vi "CANtest2.vi"() -> ()   [LabVIEW 2017]
uses:
  <vilib>/addons/Maxon Motor/EPOS2 CANopen/EPOS2 Support Files/Typedefs/EPOS2 Status Word PVM.ctl
  <vilib>/addons/Maxon Motor/EPOS2 CANopen/EPOS2 Support Files/Typedefs/EPOS2 Data Output Current.ctl
  <vilib>/addons/Maxon Motor/EPOS2 CANopen/CANopen/sbCANopenBaseClass.lvclass
  <vilib>/addons/Maxon Motor/EPOS2 CANopen/EPOS2 Support Files/Typedefs/EPOS2 Control Word PVM.ctl
  <vilib>/Platform/TimedLoop/XDataNode/timing_clust.ctl
  <vilib>/Platform/TimedLoop/XDataNode/nitl_modes.ctl
  <vilib>/Platform/TimedLoop/XDataNode/wakeup.ctl
  <vilib>/Platform/TimedLoop/XDataNode/XDataNode.xnode
  <vilib>/Platform/TimedLoop/XDataNode/XDNodeRunTimeDep.lvlib
  <vilib>/addons/Maxon Motor/EPOS2 CANopen/EPOS2 Library.lvlib
  <vilib>/addons/Maxon Motor/EPOS2 CANopen/EPOS2 Support Files/Polymorphic SubVIs/Read PDO/EPOS2 Current Mode Read.vi
  <vilib>/addons/Maxon Motor/EPOS2 CANopen/EPOS2 Support Files/Polymorphic SubVIs/Write PDO/EPOS2 Current Mode Write.vi
panel:
  out "nmotors":i32=4
  out "Velocity 2":i32[](array[numeric])
  out "Array":refnum<class "sbCANopenBaseClass.lvclass">[](array[class])
  in  "Current":i32=10
  out "Velocity":i32[](array[numeric])
  out "I32":i32
  out "Data Output 5":T1
  out "Data Output 4":T1
  out "Data Output 3":T1
  out "Data Output":T1
  out "Array 3":u8[](array[numeric])
  out "Iteration Duration 3":i64
  out "Read Late":bool
  in  "Array 2":dbl[](array[numeric])=[500.0, 600.0, 300.0, 0.0]
  out "Statusword":T2={"Ready to Switch On"=TRUE, "Switched On"=TRUE, "Operation Enable"=TRUE, "Fault"=FALSE, "Voltage Enabled"=TRUE, "Quick Stop"=TRUE, "Switch On Disable"=FALSE, "Warning"=FALSE, "Offset Current Measured"=TRUE, "Remote"=FALSE, "Target Reached"=FALSE, "Internal Limit Active"=FALSE, "Speed"=FALSE, "Reserved"=FALSE, "Refresh Cycle of Power Stage"=FALSE, "Position Reference to Home Position"=FALSE}
  out "Node":i32
  out "During Automatic":T2
  in  "STOP Final":bool
  out "Iteration Duration":i64
  in  "stop":bool
  in  "Current 2":i32(slide) scale=-1000.0..1000.0
  out "Node ID 3":u8
  in  "motor #":i32
  in  "Switch On":bool=TRUE
  in  "motor enable":i32
  in  "enable ready 2":bool
  out "Finished Late? [i-1] 3":bool
  out "Numeric 3":i32
  out "Iteration Duration 2":i64
  out "Write Late":bool
  out "Node ID\nin while loop 2":u8
  out "Node ID\nin while loop":u8
  out "for 1":i32
  # "reading purposes"
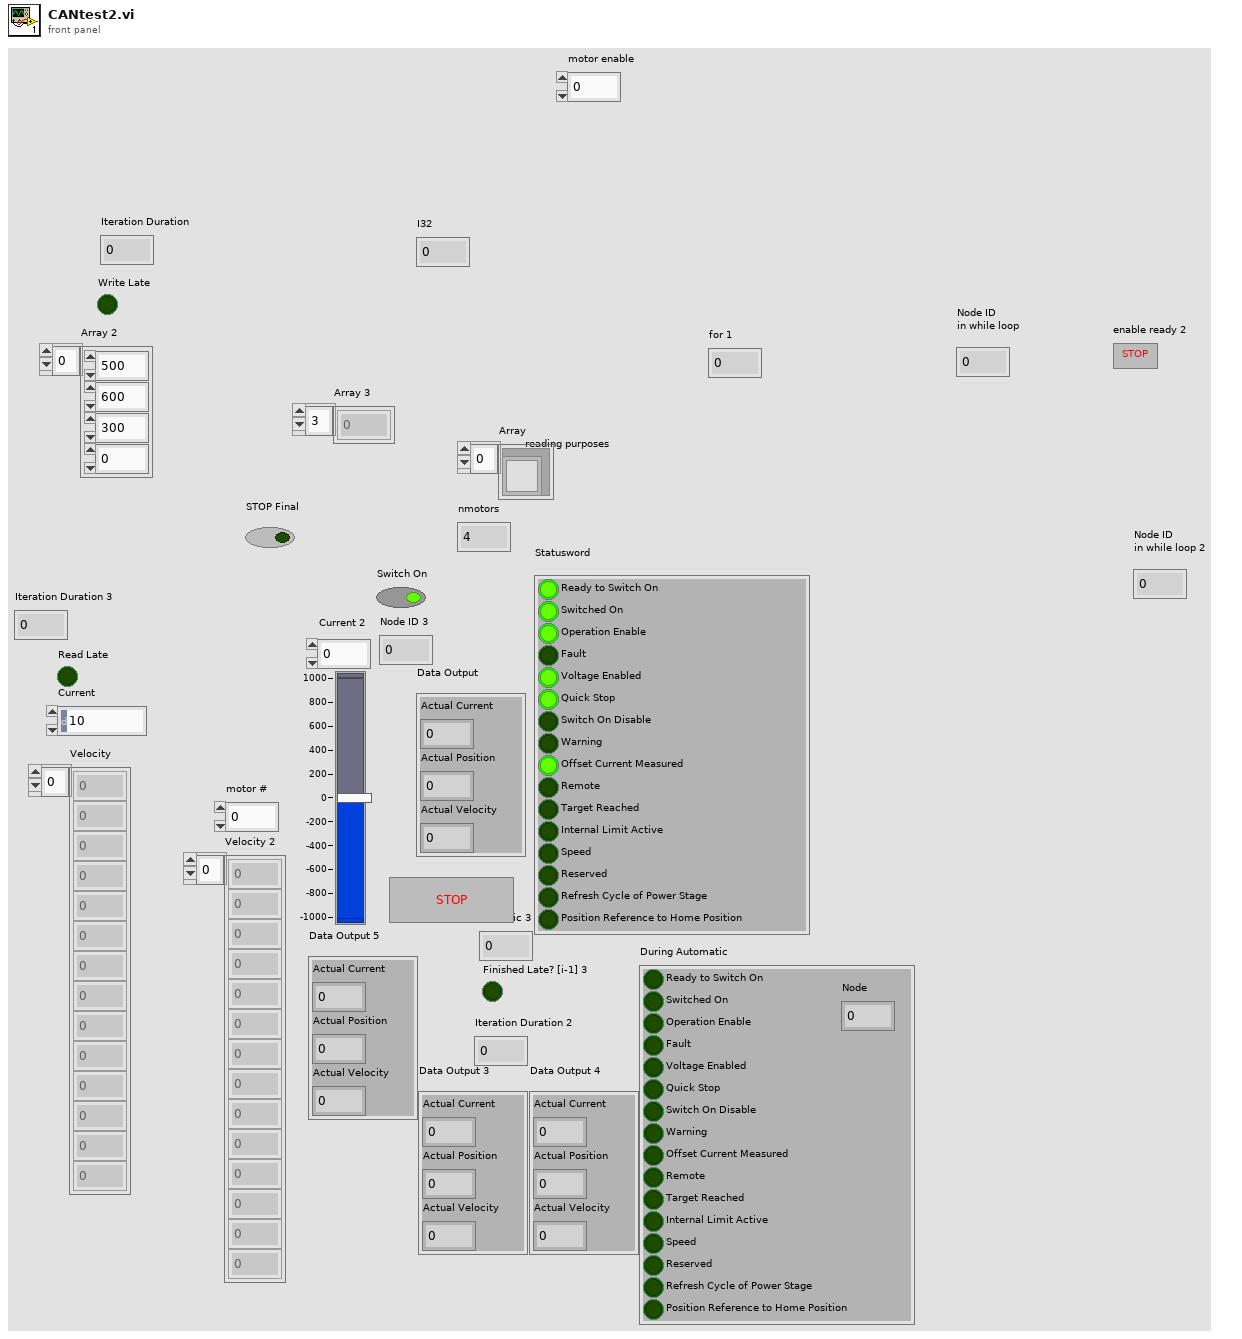
[diagram p1: front panel]
types:
  T1 = typedef "EPOS2 Library.lvlib/EPOS2 Data Output Current.ctl" = cluster{"Actual Current":i16, "Actual Position":i32, "Actual Velocity":i32}
  T2 = typedef "EPOS2 Library.lvlib/EPOS2 Status Word PVM.ctl" = cluster{"Ready to Switch On":bool, "Switched On":bool, "Operation Enable":bool, "Fault":bool, "Voltage Enabled":bool, "Quick Stop":bool, "Switch On Disable":bool, "Warning":bool, "Offset Current Measured":bool, "Remote":bool, "Target Reached":bool, "Internal Limit Active":bool, "Speed":bool, "Reserved":bool, "Refresh Cycle of Power Stage":bool, "Position Reference to Home Position":bool}
  T3 = typedef "XDNodeRunTimeDep.lvlib/timing_clust.ctl" = cluster{"Expected End [f-1]":u64, "Actual End [f-1]":u64, "Finished Late? [f-1]":bool, "Expected End [i-1]":u64, "Actual End [i-1]":u64, "Finished Late? [i-1]":bool, "Expected Start [i]":u64, "Actual Start [i]":u64, "Expected Start [f]":u64, "Actual Start [f]":u64, "Source Name":string, "Structure Name":string, "Period":i64, "Deadline":i64, "Offset":i64, "Start":i64, "Priority":i32, "Timeout":i32, "Mode":T4, "Wakeup Reason":T5, "Error":errorcluster, "Source Type":string, "Secondary Source Type":string, "Global End Time":u64, "Global Start Time":u64, "Frame Duration":u64, "Iteration Duration":u64, "Assigned CPU":i32, "I/O Scan Engine Mode":u32}
  T4 = typedef "XDNodeRunTimeDep.lvlib/nitl_modes.ctl" = enum32{"No Change", "Process missed periods, maintain original phase", "Discard missed periods, maintain original phase", "Process missed periods, ignore original phase", "Discard missed periods, ignore original phase"}
  T5 = typedef "XDNodeRunTimeDep.lvlib/wakeup.ctl" = enum32{"Normal", "Aborted", "Asynchronous wakeup", "Timing source error", "Timed loop error", "Timeout"}
  T6 = typedef "EPOS2 Library.lvlib/EPOS2 Control Word PVM.ctl" = cluster{"Switch On":bool, "Enable Voltage":bool, "Quick Stop":bool, "Enable Operation":bool, "Reserved 0":bool, "Reserved 1":bool, "Reserved 2":bool, "Fault Reset":bool, "Halt":bool}
  T7 = cluster{"[0]":bool, "[1]":bool, "[2]":bool, "[3]":bool, "[4]":bool, "[5]":bool, "[6]":bool, "[7]":bool, "[8]":bool, "[9]":bool, "[10]":bool, "[11]":bool, "[12]":bool, "[13]":bool, "[14]":bool, "[15]":bool}
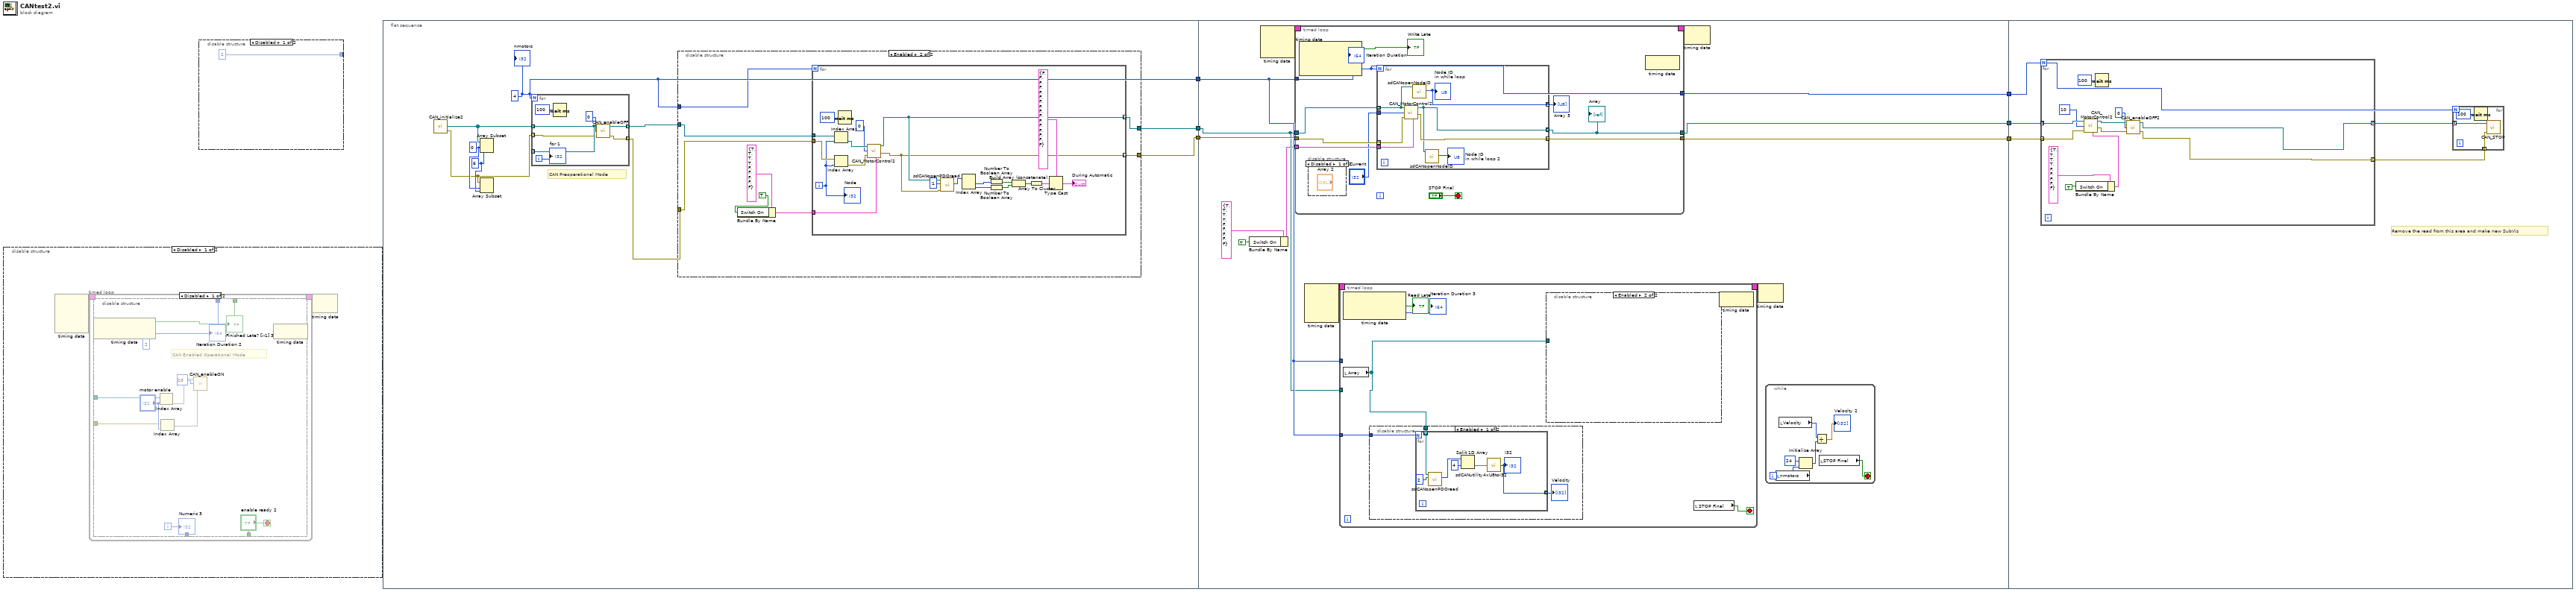
[diagram p0: block diagram]
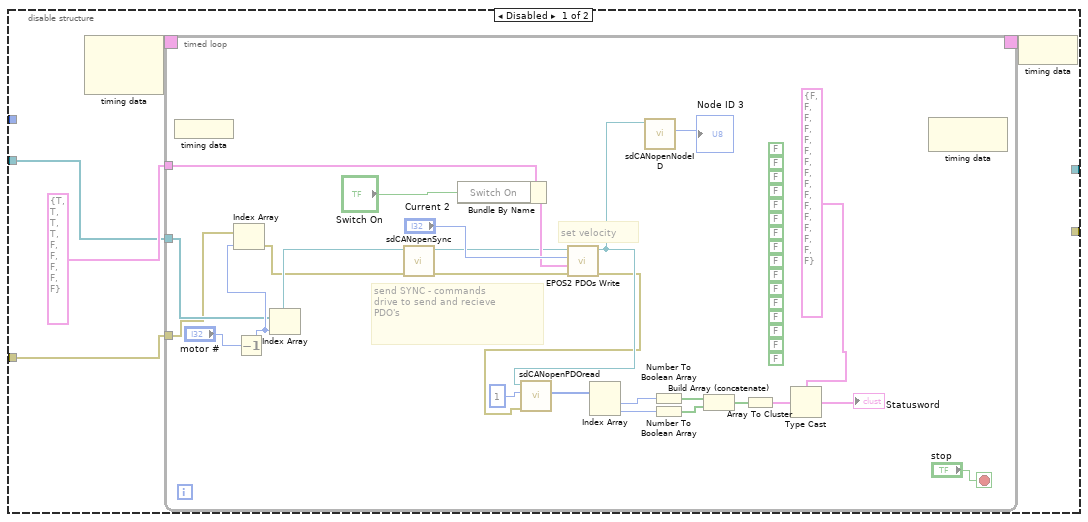
[diagram p5: hidden frame]
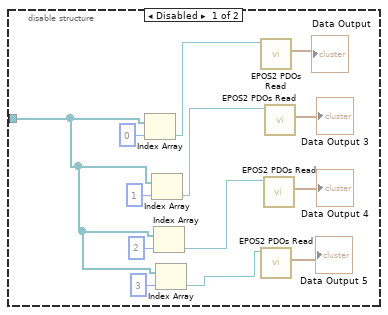
[diagram p7: hidden frame]
diagram:
  n1 = disable-structure shown="Disabled" {
    frame Disabled {
      n2 = node-c288() -> (w8:T3)  [unwired: 4 in]
      n3 = timed-loop {
        timing: w8 -> [_]
        timing-out: [_] -> w7
        i -> [w10]
        stop <- w12 stop-if-true
        n4 = node-c288() -> (w11:bool, w9:i64)  [unwired: 1 in]
        n5 = disable-structure shown="Disabled" {
          disable-tunnel: ["enable ready 2" _] -> w12
          disable-tunnel: w11 -> [w21 _]
          disable-tunnel: w10 -> [w20 _]
          disable-tunnel: w9 -> [w19 _]
          disable-tunnel: _ -> [w16 _]
          disable-tunnel: _ -> [w14 _]
          frame Disabled {
            (unwired) 2
            # "CAN Enabled Operational Mode"
            n6 = Index Array(array=w16, index="motor enable") -> (element=w18)
            n7 = Index Array(array=w14, index="motor enable") -> (element=w17)
            n8 = call "CAN_enableON.vi"("error in (no error)"=w17, "Current"=20, "sbCANopenBaseClass in"=w18) -> ()  [unwired: 1 in, 2 out]
            "Finished Late? [i-1] 3" <- w21
            "Numeric 3" <- w20
            "Iteration Duration 2" <- w19
          }
          frame Enabled {
          }
        }
        n9 = node-c288() -> ()  [unwired: 1 in, 1 out]
      }
      n10 = node-c288(w7) -> ()  [unwired: 1 out]
    }
    frame Enabled {
    }
  }
  n11 = disable-structure shown="Disabled" {
    disable-tunnel: [2 _] -> _
    frame Disabled {
    }
    frame Enabled {
    }
  }
  n12 = flat-sequence {
    tunnel: [w37] -> w5
    tunnel: [w36] -> w4
    tunnel: [w30] -> w3
    tunnel: [w121] -> w6
    tunnel: w5 -> [w111]
    tunnel: w4 -> [w117]
    tunnel: w3 -> [w112]
    tunnel: [w118] -> w2
    tunnel: [w116] -> w1
    tunnel: w6 -> [w190]
    tunnel: w2 -> [w189]
    tunnel: w1 -> [w188]
    frame #0 {
      w30 = 4
      w33 = 6 ("length")
      w34 = 0 ("index")
      # "CAN Preoperational Mode"
      n13 = call "CAN_initialize2.vi"() -> ("Array 2"=w31:errorcluster[], "Array"=w32:refnum<class "sbCANopenBaseClass.lvclass">[])  [unwired: 3 in, 1 out]
      n14 = Array Subset(array=w32, index=w34, length=w33) -> ()  [unwired: 1 out]
      n15 = Array Subset(array=w31, index=w34, length=w33) -> ()  [unwired: 1 out]
      n16 = for {
        N: w30 -> [_]
        tunnel: [w106] -> _ mode=indexing
        tunnel: [w107] -> w38 mode=indexing
        tunnel: w32 -> [w106] mode=indexing
        tunnel: w31 -> [w105] mode=indexing
        tunnel: [w102] -> w35 mode=indexing
        i -> [w103]
        n17 = Wait (ms)(milliseconds to wait=u32 100) -> ()  [unwired: 1 out]
        n18 = call "CAN_enableOFF.vi"("error in (no error)"=w105, "Current"=0, "sbCANopenBaseClass in"=w106) -> ("error out"=w107:errorcluster, "CANopen Session Out"=w102:refnum<class "sbCANopenBaseClass.lvclass">)  [unwired: 1 in]
        "for 1" <- w103
      }
      n19 = disable-structure shown="Enabled" {
        disable-tunnel: w35 -> [w40 w80]
        disable-tunnel: w38 -> [w39 w79]
        disable-tunnel: w30 -> [_ w81]
        disable-tunnel: [_ w75] -> w37
        disable-tunnel: [_ w74] -> w36
        frame Disabled {
          n20 = node-c288() -> (w43:T3)  [unwired: 2 out]
          n21 = timed-loop {
            timing: w43 -> [_]
            timing-out: [_] -> w42
            tunnel: T6 {"Switch On"=TRUE, "Enable Voltage"=TRUE, "Quick Stop"=TRUE, "Enable Operation"=TRUE, "Reserved 0"=FALSE, "Reserved 1"=FALSE, "Reserved 2"=FALSE, "Fault Reset"=FALSE, "Halt"=FALSE} ("Control Word") -> [w67]
            tunnel: w40 -> [w58]
            tunnel: w39 -> [w57]
            stop <- "stop" stop-if-true
            (unwired) FALSE ("Ready to Switch On")
            (unwired) FALSE ("Switched On")
            (unwired) FALSE ("Operation Enable")
            (unwired) FALSE ("Fault")
            (unwired) FALSE ("Voltage Enabled")
            (unwired) FALSE ("Quick Stop")
            (unwired) FALSE ("Switch On Disable")
            (unwired) FALSE ("Warning")
            (unwired) FALSE ("Offset Current Measured")
            (unwired) FALSE ("Remote")
            (unwired) FALSE ("Target Reached")
            (unwired) FALSE ("Internal Limit Active")
            (unwired) FALSE ("Speed")
            (unwired) FALSE ("Reserved")
            (unwired) FALSE ("Refresh Cycle of Power Stage")
            (unwired) FALSE ("Position Reference to Home Position")
            # "set velocity"
            # "send SYNC - commands\ndrive to send and recieve\nPDO's"
            n22 = node-c288() -> ()  [unwired: 1 out]
            n23 = Decrement(x="motor #") -> (x-1=w60:i32)
            n24 = Index Array(array=w57, index=w60) -> (element=w59:errorcluster)
            n25 = Index Array(array=w58, index=w60) -> (element=w63:refnum<class "sbCANopenBaseClass.lvclass">)
            n26 = call-dynamic "sdCANopenSync.vi"("error in (no error)"=w59, "sbCANopenBaseClass in"=w63) -> ("error out"=w69:errorcluster, "sbCANopenBaseClass out"=w65:refnum<class "sbCANopenBaseClass.lvclass">)  [unwired: 8 in]
            n27 = Bundle By Name(cluster=w67, "Switch On"="Switch On") -> (w66:T6)
            n28 = call-poly <vilib>:"EPOS2 PDOs Write.vi"("error in"=w69, "Control Word"=w66, "Current"="Current 2", "CANopen Session In"=w65) -> ("error out"=w46:errorcluster, "CANopen Session Out"=w47:refnum<class "sbCANopenBaseClass.lvclass">)  [unwired: 6 in]
            n29 = call-dynamic "sdCANopenPDOread.vi"("error in (no error)"=w46, "PDO Number"=u8 1, "sbCANopenBaseClass in"=w47) -> ("Data"=w55:u8[])  [unwired: 6 in, 2 out]
            n30 = Index Array(array=w55) -> (element #1=w52:u8, element #2=w53:u8)  [unwired: 2 in]
            n31 = call-dynamic "sdCANopenNodeID.vi"("sbCANopenBaseClass in"=w47) -> ("Node ID"=→"Node ID 3":u8)  [unwired: 9 in, 1 out]
            n32 = Number To Boolean Array(number=w52) -> (Boolean array=w49:bool[])
            n33 = Number To Boolean Array(number=w53) -> (Boolean array=w50:bool[])
            n34 = Build Array (concatenate)(w49, w50) -> (w51:bool[])
            n35 = Array To Cluster(array=w51) -> (cluster=w54:T7)
            n36 = Type Cast(type=T2 {"Ready to Switch On"=FALSE, "Switched On"=FALSE, "Operation Enable"=FALSE, "Fault"=FALSE, "Voltage Enabled"=FALSE, "Quick Stop"=FALSE, "Switch On Disable"=FALSE, "Warning"=FALSE, "Offset Current Measured"=FALSE, "Remote"=FALSE, "Target Reached"=FALSE, "Internal Limit Active"=FALSE, "Speed"=FALSE, "Reserved"=FALSE, "Refresh Cycle of Power Stage"=FALSE, "Position Reference to Home Position"=FALSE} ("IPM Statusword 2"), x=w54) -> (*(type *) &x=→"Statusword":T2)
            n37 = node-c288() -> ()  [unwired: 2 out]
          }
          n38 = node-c288(w42) -> ()
        }
        frame Enabled {
          n39 = Bundle By Name(cluster=T6 {"Switch On"=TRUE, "Enable Voltage"=TRUE, "Quick Stop"=TRUE, "Enable Operation"=TRUE, "Reserved 0"=FALSE, "Reserved 1"=FALSE, "Reserved 2"=FALSE, "Fault Reset"=FALSE, "Halt"=FALSE} ("Control Word"), "Switch On"=TRUE) -> (w76:T6)
          n40 = for {
            N: w81 -> [_]
            tunnel: w80 -> [w101]
            tunnel: w79 -> [w99]
            tunnel: [w87] -> w75 mode=indexing
            tunnel: [w85] -> w74 mode=indexing
            tunnel: w76 -> [w82]
            i -> [w95]
            n41 = Index Array(array=w99, index=w95) -> (element=w98:errorcluster)
            n42 = Index Array(array=w101, index=w95) -> (element=w100:refnum<class "sbCANopenBaseClass.lvclass">)
            n43 = Wait (ms)(milliseconds to wait=u32 100) -> ()  [unwired: 1 out]
            n44 = call "CAN_MotorControl2.vi"("output cluster"=w82, "sbCANopenBaseClass in"=w100, "Current"=0, "error in (no error)"=w98) -> ("CANopen Session Out"=w87:refnum<class "sbCANopenBaseClass.lvclass">, "error out"=w85:errorcluster)  [unwired: 2 in]
            n45 = call-dynamic "sdCANopenPDOread.vi"("error in (no error)"=w85, "PDO Number"=u8 1, "sbCANopenBaseClass in"=w87) -> ("Data"=w84:u8[])  [unwired: 6 in, 2 out]
            n46 = Index Array(array=w84) -> (element #1=w91:u8, element #2=w90:u8)  [unwired: 2 in]
            n47 = Number To Boolean Array(number=w91) -> (Boolean array=w94:bool[])
            n48 = Number To Boolean Array(number=w90) -> (Boolean array=w93:bool[])
            n49 = Build Array (concatenate)(w94, w93) -> (w92:bool[])
            n50 = Array To Cluster(array=w92) -> (cluster=w89:T7)
            n51 = Type Cast(type=T2 {"Ready to Switch On"=FALSE, "Switched On"=FALSE, "Operation Enable"=FALSE, "Fault"=FALSE, "Voltage Enabled"=FALSE, "Quick Stop"=FALSE, "Switch On Disable"=FALSE, "Warning"=FALSE, "Offset Current Measured"=FALSE, "Remote"=FALSE, "Target Reached"=FALSE, "Internal Limit Active"=FALSE, "Speed"=FALSE, "Reserved"=FALSE, "Refresh Cycle of Power Stage"=FALSE, "Position Reference to Home Position"=FALSE} ("IPM Statusword 2"), x=w89) -> (*(type *) &x=→"During Automatic":T2)
            "Node" <- w95
          }
        }
      }
      "nmotors" <- w30
    }
    frame #1 {
      n52 = Bundle By Name(cluster=T6 {"Switch On"=TRUE, "Enable Voltage"=TRUE, "Quick Stop"=TRUE, "Enable Operation"=TRUE, "Reserved 0"=FALSE, "Reserved 1"=FALSE, "Reserved 2"=FALSE, "Fault Reset"=FALSE, "Halt"=FALSE} ("Control Word"), "Switch On"=TRUE) -> (w113:T6)
      n53 = node-c288() -> (w120:T3)  [unwired: 3 in]
      n54 = timed-loop {
        tunnel: w117 -> [w169]
        tunnel: [w166] -> w121
        timing: w120 -> [_]
        timing-out: [_] -> w119
        tunnel: w112 -> [w161]
        tunnel: [w161] -> w118
        tunnel: w113 -> [w164]
        tunnel: w111 -> [w170]
        tunnel: [w165] -> w116
        stop <- "STOP Final" stop-if-true
        n55 = node-c288() -> (→"Write Late":bool, →"Iteration Duration":i64)  [unwired: 1 in, 2 out]
        n56 = disable-structure shown="Disabled" {
          frame Disabled {
          }
          frame Enabled {
          }
        }
        n57 = for {
          N: w161 -> [_]
          tunnel: [w179] -> w165 mode=indexing
          tunnel: [w180] -> w166 mode=indexing
          tunnel: w170 -> [w182] mode=indexing
          tunnel: w169 -> [w183] mode=indexing
          tunnel: w164 -> [w178]
          tunnel: [w177] -> w163 mode=indexing
          tunnel: "Current" -> [w176]
          n58 = call "CAN_MotorControl2.vi"("output cluster"=w178, "sbCANopenBaseClass in"=w182, "Current"=w176, "error in (no error)"=w183) -> ("CANopen Session Out"=w179:refnum<class "sbCANopenBaseClass.lvclass">, "error out"=w180:errorcluster)  [unwired: 2 in]
          n59 = call-dynamic "sdCANopenNodeID.vi"("sbCANopenBaseClass in"=w182) -> ("Node ID"=w177:u8)  [unwired: 9 in, 1 out]
          "Node ID\nin while loop" <- w177
          n60 = call-dynamic "sdCANopenNodeID.vi"("sbCANopenBaseClass in"=w179) -> ("Node ID"=→"Node ID\nin while loop 2":u8)  [unwired: 9 in, 1 out]
        }
        "Array 3" <- w163
        "Array" <- w165
        n61 = node-c288() -> ()  [unwired: 1 in, 1 out]
      }
      n62 = node-c288() -> (w110:T3)  [unwired: 4 in]
      n63 = timed-loop {
        timing: w110 -> [_]
        timing-out: [_] -> w109
        tunnel: w112 -> [_]
        tunnel: w111 -> [_]
        tunnel: w112 -> [w129]
        stop <- w132 stop-if-true
        n64 = node-c288() -> (→"Read Late":bool, →"Iteration Duration 3":i64)  [unwired: 1 in, 1 out]
        n65 = local read "Array"() -> (w128:refnum<class "sbCANopenBaseClass.lvclass">[])
        n66 = disable-structure shown="Enabled" {
          disable-tunnel: w128 -> [w135 _]
          disable-tunnel: w129 -> [w133 _]
          frame Enabled {
            n67 = for {
              N: w133 -> [_]
              tunnel: w135 -> [w137] mode=indexing
              tunnel: [w138] -> w134 mode=indexing
              n68 = call-dynamic "sdCANopenPDOread.vi"("PDO Number"=u8 2, "sbCANopenBaseClass in"=w137) -> ("Data"=w139:u8[])  [unwired: 7 in, 2 out]
              n69 = Split 1D Array(array=w139, index=4) -> (second subarray=w136:u8[])  [unwired: 1 out]
              n70 = call <vilib>:"sdCANutility4xU8toI32.vi"("Array 4 U8"=w136) -> ("I32"=w138:i32)
              "I32" <- w138
            }
            "Velocity" <- w134
          }
          frame Disabled {
          }
        }
        n71 = disable-structure shown="Enabled" {
          disable-tunnel: w128 -> [w142 _]
          frame Disabled {
            n72 = Index Array(array=w142, index=0) -> (element=w150:refnum<class "sbCANopenBaseClass.lvclass">)
            n73 = Index Array(array=w142, index=1) -> (element=w149:refnum<class "sbCANopenBaseClass.lvclass">)
            n74 = Index Array(array=w142, index=2) -> (element=w148:refnum<class "sbCANopenBaseClass.lvclass">)
            n75 = Index Array(array=w142, index=3) -> (element=w147:refnum<class "sbCANopenBaseClass.lvclass">)
            n76 = call-poly <vilib>:"EPOS2 PDOs Read.vi"("CANopen Session In"=w150) -> ("Data Output"=→"Data Output":T1)  [unwired: 7 in, 3 out]
            n77 = call-poly <vilib>:"EPOS2 PDOs Read.vi"("CANopen Session In"=w147) -> ("Data Output"=→"Data Output 5":T1)  [unwired: 7 in, 3 out]
            n78 = call-poly <vilib>:"EPOS2 PDOs Read.vi"("CANopen Session In"=w148) -> ("Data Output"=→"Data Output 4":T1)  [unwired: 7 in, 3 out]
            n79 = call-poly <vilib>:"EPOS2 PDOs Read.vi"("CANopen Session In"=w149) -> ("Data Output"=→"Data Output 3":T1)  [unwired: 7 in, 3 out]
          }
          frame Enabled {
          }
        }
        n80 = local read "STOP Final"() -> (w132:bool)
        n81 = node-c288() -> ()  [unwired: 1 in, 1 out]
      }
      n82 = node-c288(w119) -> ()  [unwired: 1 out]
      n83 = node-c288(w109) -> ()  [unwired: 1 out]
      n84 = while {
        stop <- w127 stop-if-true
        n85 = local read "nmotors"() -> (w124:i32)
        n86 = local read "Velocity"() -> (w126:i32[])
        n87 = Initialize Array(24 ("element"), w124) -> (w122:i32[])
        n88 = Divide(x=w126, y=w122) -> (x/y=→"Velocity 2":dbl[])
        n89 = local read "STOP Final"() -> (w127:bool)
      }
    }
    frame #2 {
      # "Remove the read from this area and make new SubVis"
      n90 = for {
        N: w189 -> [_]
        tunnel: w190 -> [w203] mode=indexing
        tunnel: w188 -> [w204] mode=indexing
        tunnel: [w196] -> w187 mode=indexing
        tunnel: [w195] -> w186 mode=indexing
        n91 = Bundle By Name(cluster=T6 {"Switch On"=TRUE, "Enable Voltage"=TRUE, "Quick Stop"=TRUE, "Enable Operation"=TRUE, "Reserved 0"=FALSE, "Reserved 1"=FALSE, "Reserved 2"=FALSE, "Fault Reset"=FALSE, "Halt"=FALSE} ("Control Word"), "Switch On"=TRUE) -> (w200:T6)
        n92 = call "CAN_MotorControl2.vi"("output cluster"=w200, "sbCANopenBaseClass in"=w204, "Current"=10, "error in (no error)"=w203) -> ("CANopen Session Out"=w199:refnum<class "sbCANopenBaseClass.lvclass">, "error out"=w198:errorcluster)  [unwired: 2 in]
        n93 = Wait (ms)(milliseconds to wait=u32 100) -> ()  [unwired: 1 out]
        n94 = call "CAN_enableOFF2.vi"("error in (no error)"=w198, "Current"=0, "sbCANopenBaseClass in"=w199) -> ("error out"=w195:errorcluster, "CANopen Session Out"=w196:refnum<class "sbCANopenBaseClass.lvclass">)  [unwired: 1 in]
      }
      n95 = for {
        N: w189 -> [_]
        tunnel: w187 -> [w192] mode=indexing
        tunnel: w186 -> [w191] mode=indexing
        n96 = Wait (ms)(milliseconds to wait=u32 100) -> ()  [unwired: 1 out]
        n97 = call "CAN_STOP.vi"("error in"=w191, "CANopen Session In"=w192) -> ()  [unwired: 3 in, 1 out]
      }
    }
  }
